vi "Main.vi"() -> ()   [LabVIEW 2018]
doc: "This Continuous Measurement sample project is based on the Queued Message Handler template.\n\nThe Event Handling Loop generates messages based on user interface actions.\n\nThe Message Handling Loop processes messages generated by the Event Handling Loop, or by other messages. There are also Acquisition and Logging message handling loop subVIs, and a chart updating loop."
uses:
  Settings/Settings.ctl
  Acquisition/Hardware Configuration.ctl
  Acquisition/Signal Type.ctl
  Logging/Logging Configuration.ctl
  controls/UI Data.ctl
  controls/UI State.ctl
  support/Message Queue/Enqueue Message (Single).vi
  controls/ExitGlobal.vi
  support/Message Queue/Enqueue Message (Array).vi
  <vilib>/Utility/error.llb/Error Cluster From Error Code.vi
  <vilib>/ErrorRing/Error Ring.xnode
  Acquisition/Acquisition.lvlib
  Logging/Logging.lvlib
  Settings/Settings.lvlib
  support/User Event - Stop/User Event - Stop.lvlib
  support/Message Queue/Message Queue.lvlib
  Settings/Settings Dialog.vi
panel:
  out "Data":waveform(dbl)[](graph)
  out "Zero run":bool
  in  "Zero run?":bool
  out "Max writing time to a file [min]":dbl
  out "Test time zero run [s]":dbl
  out "Test time [min]":dbl
  in  "Start":bool
  in  "Stop":bool
  in  "Settings":bool
  out "Status":string
  in  "Exit":bool
  out "Log File Offsite Path":path
  out "Project code":string
  out "Offsite storage?":bool
  out "Log File Path":path
  # "Continuous Measurement Data Logger"
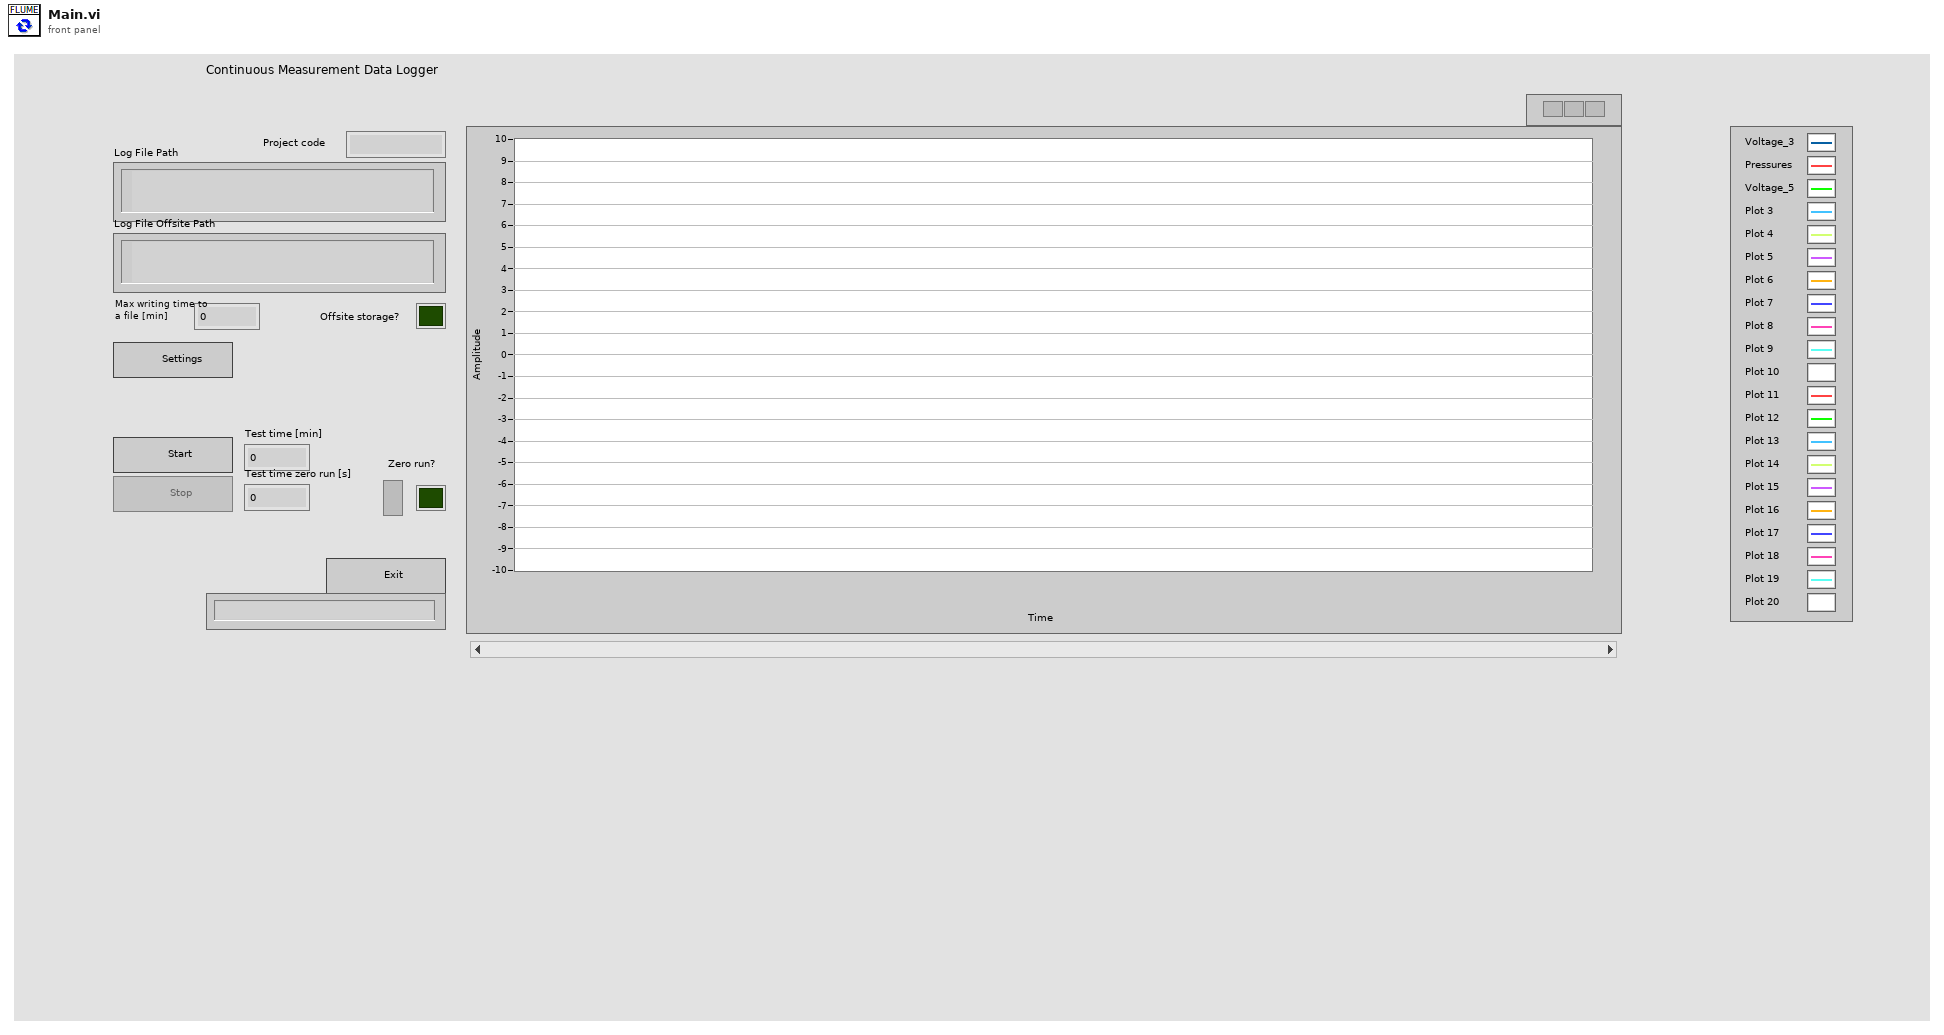
[diagram p1: front panel]
types:
  T1 = cluster{"Offsite storage?":bool, "Test time [s]":dbl, "Test time zero run [s] ":dbl, "Max writing time to a file [min]":dbl, "Zero run":bool}
  T2 = typedef "UI State.ctl" = enum16{"Idle", "Acquiring and Logging", "Waiting for Exit", "Waiting for Exit (Acq Stopped)", "Waiting for Exit (Log Stopped)", "Waiting for Stop", "Waiting for Stop (Acq Stopped)", "Waiting for Stop (Log Stopped)"}
  T3 = typedef "UI Data.ctl" = cluster{"Start Ref":refnum<vi>, "Stop Ref":refnum<vi>, "Settings Ref":refnum<vi>, "Exit Ref":refnum<vi>, "Status Ref":refnum<vi>, "Data Ref":refnum<vi>, "Zero run Ref":refnum<vi>}
  T4 = typedef "Settings.lvlib/Settings.ctl" = cluster{"Hardware Configuration":T5, "Logging Configuration":T7, "Timers":cluster{"Offsite storage?":bool, "Test time [s]":dbl, "Test time zero run [s] ":dbl, "Max writing time to a file [min]":dbl, "Zero run":bool}}
  T5 = typedef "Acquisition.lvlib/Hardware Configuration.ctl" = cluster{"DAQ1":string, "Signal Type 1":T6, "DAQ2":string, "Signal Type 2":T6, "DAQ3":string, "Signal Type 3":T6}
  T6 = typedef "Acquisition.lvlib/Signal Type.ctl" = enum16{"DAQ simulated", "Sine and square wave", "Sine wave"}
  T7 = typedef "Logging.lvlib/Logging Configuration.ctl" = cluster{"Log File Base Path":path, "TDMS File Reference":refnum<k34>, "Log File Offsite Path":path, "Project code":string, "Bin File Reference":refnum<k34>}
  T8 = typedef "Message Queue.lvlib/All Message Queues.ctl" = cluster{"UI":refnum<queue>, "Acquisition":refnum<queue>, "Logging":refnum<queue>, "Bin Logging":refnum<queue>, "Time":refnum<queue>}
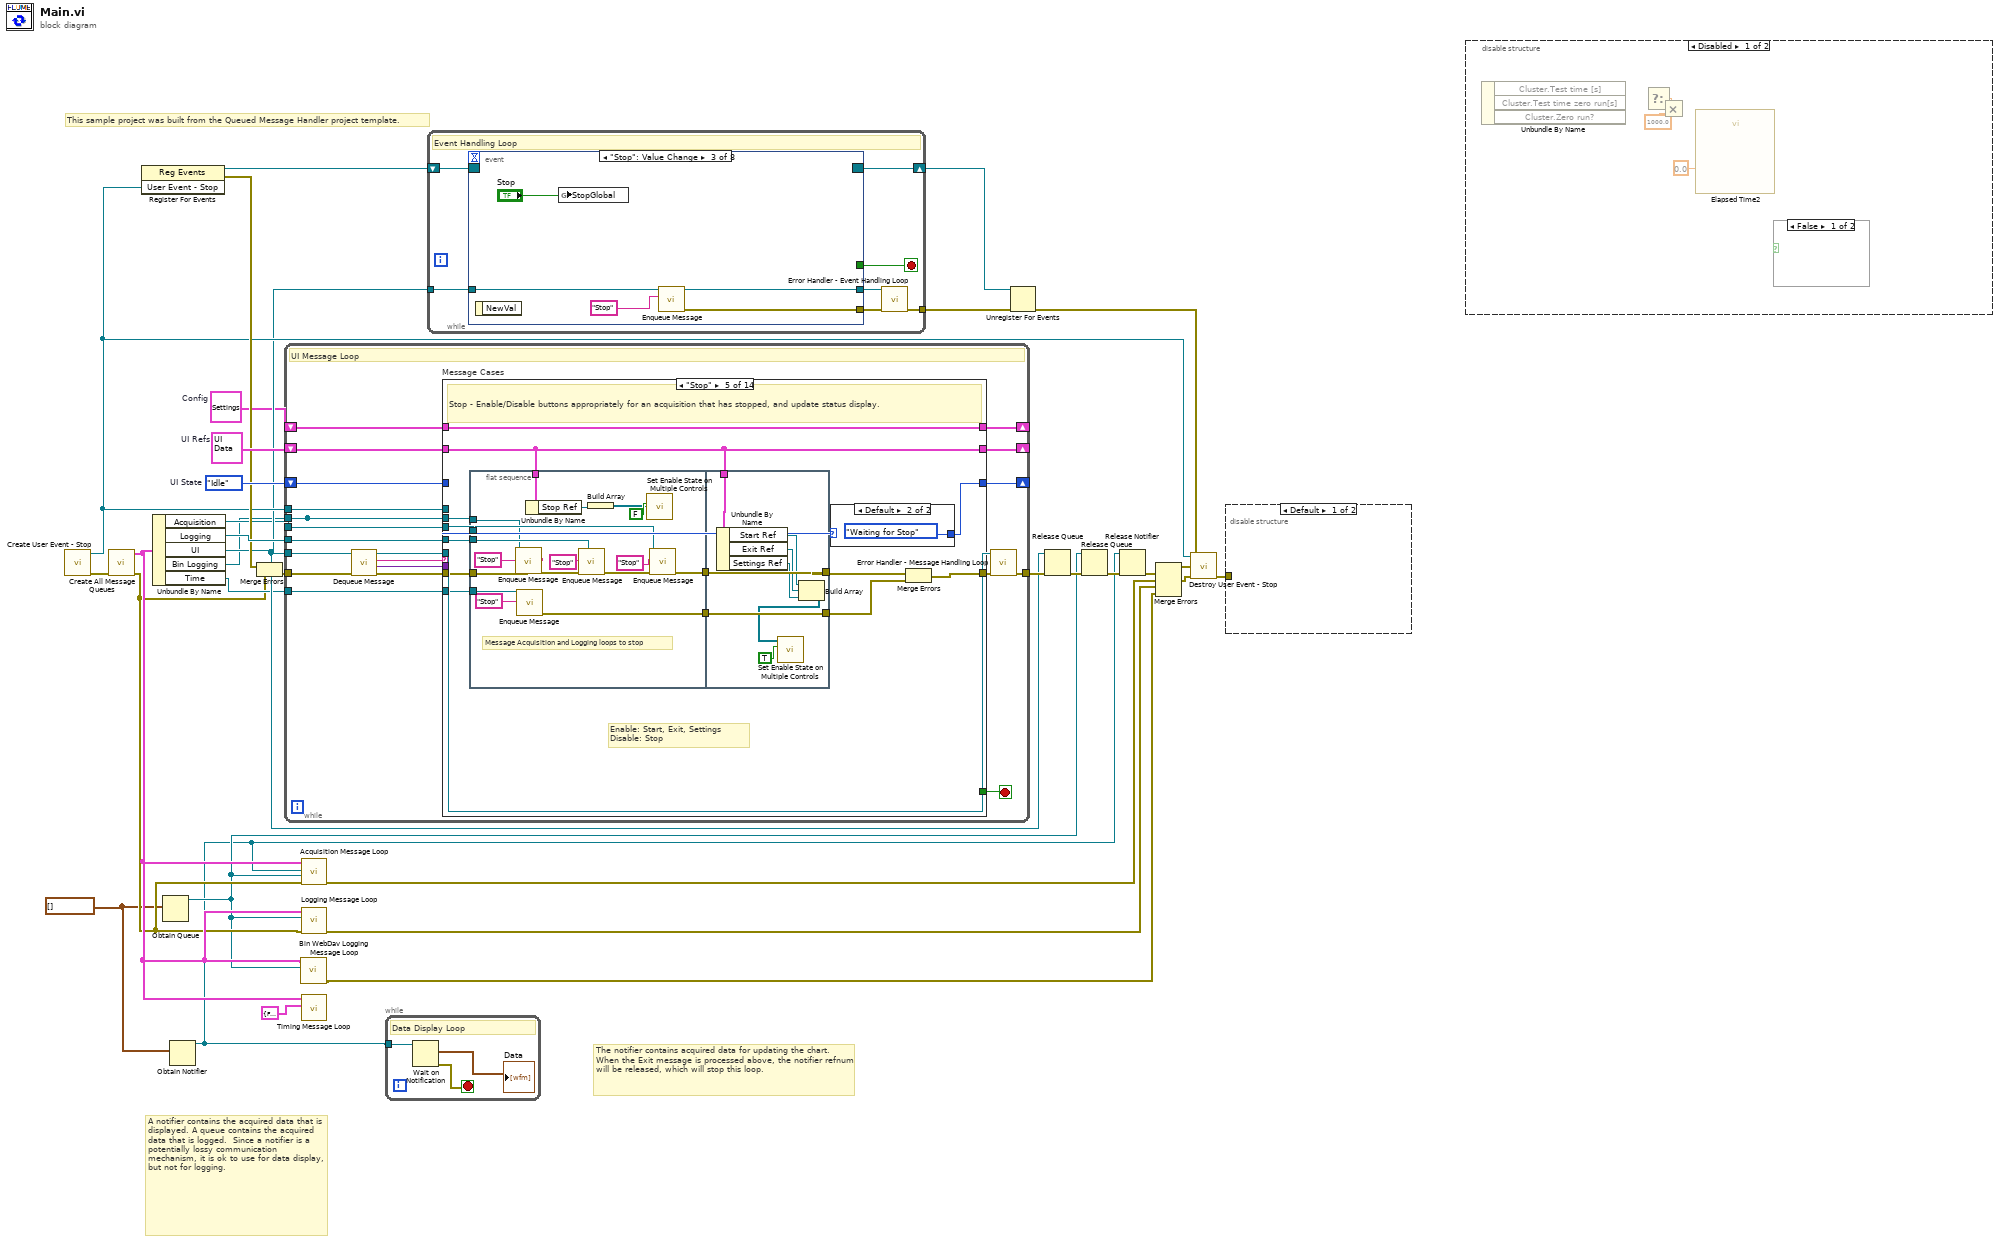
[diagram p0: block diagram]
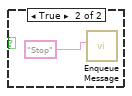
[diagram p2: hidden frame]
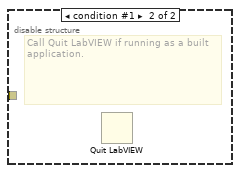
[diagram p4: hidden frame]
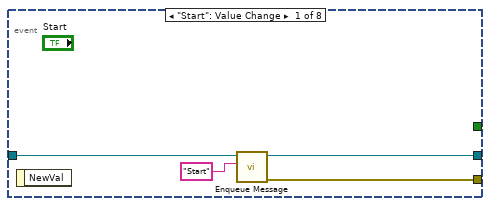
[diagram p5: hidden frame]
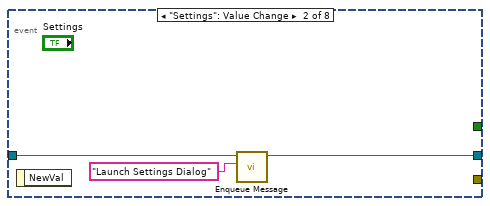
[diagram p6: hidden frame]
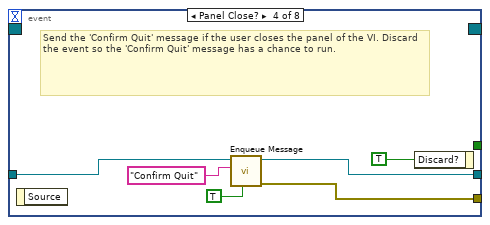
[diagram p7: hidden frame]
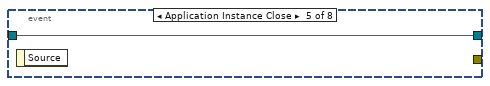
[diagram p8: hidden frame]
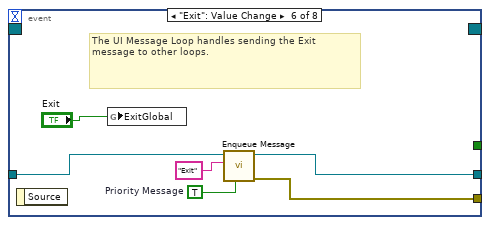
[diagram p9: hidden frame]
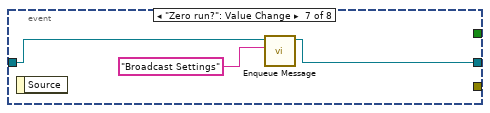
[diagram p10: hidden frame]
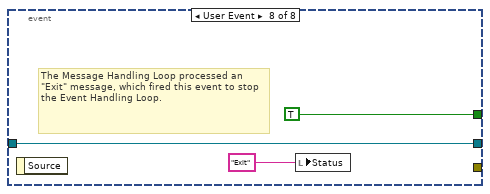
[diagram p11: hidden frame]
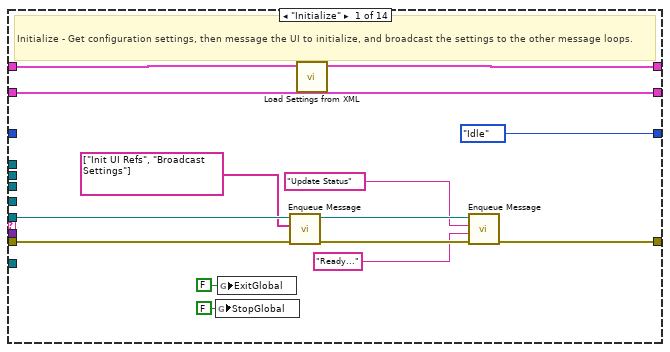
[diagram p12: hidden frame]
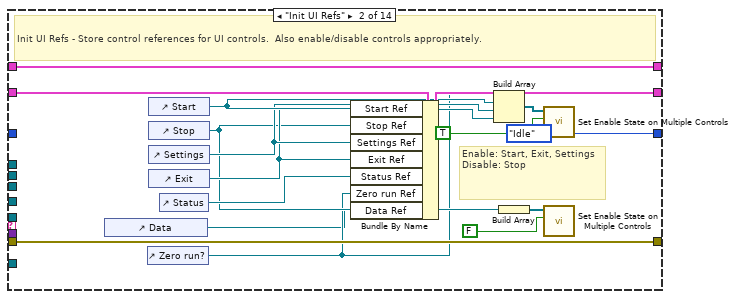
[diagram p13: hidden frame]
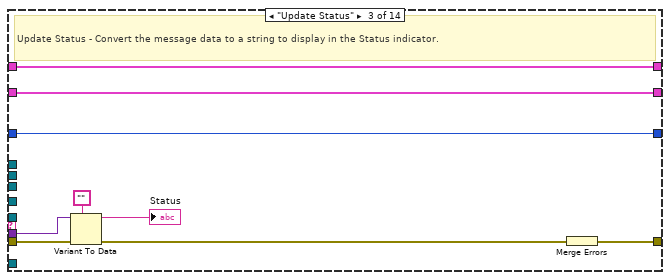
[diagram p14: hidden frame]
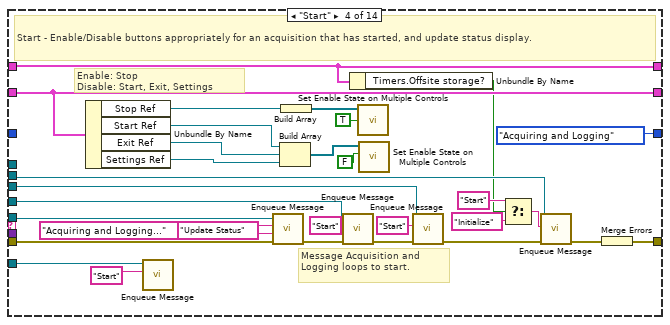
[diagram p15: hidden frame]
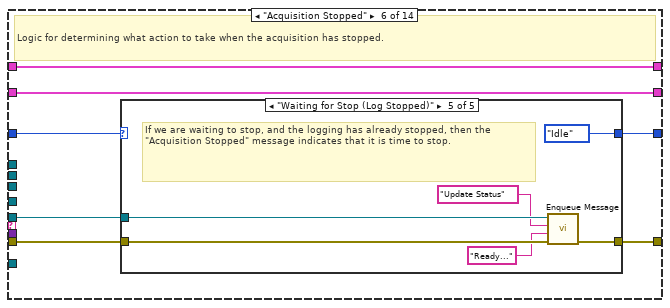
[diagram p17: hidden frame]
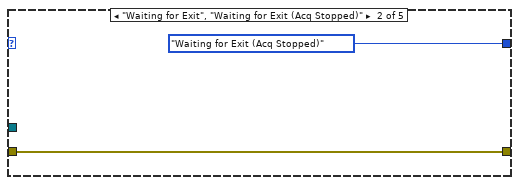
[diagram p19: hidden frame]
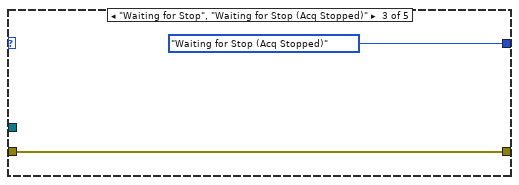
[diagram p20: hidden frame]
diagram:
  w2 = waveform(dbl)[] []
  w25 = UI_State."Idle"  # UI State
  w27 = T3 {"Start Ref"=refnum, "Stop Ref"=refnum, "Settings Ref"=refnum, "Exit Ref"=refnum, "Status Ref"=refnum, "Data Ref"=refnum, "Zero run Ref"=refnum}  # UI Refs
  w12 = T4 {"Hardware Configuration"={"DAQ1"="", "Signal Type 1"=enum."DAQ simulated", "DAQ2"="", "Signal Type 2"=enum."DAQ simulated", "DAQ3"="", "Signal Type 3"=enum."DAQ simulated"}, "Logging Configuration"={"Log File Base Path"=path "", "TDMS File Reference"=refnum, "Log File Offsite Path"=path "", "Project code"="", "Bin File Reference"=refnum}, "Timers"={"Offsite storage?"=FALSE, "Test time [s]"=10.0, "Test time zero run [s] "=180.0, "Max writing time to a file [min]"=30.0, "Zero run"=FALSE}}  # Config
  # "This sample project was built from the Queued Message Handler project template."
  # "A notifier contains the acquired data that is displayed. A queue contains the acquired data that is logged.  Since a notifier is a potentially lossy communication mechanism, it is ok to use for data display, but not for logging."
  # "The notifier contains acquired data for updating the chart. When the Exit message is processed above, the notifier refnum will be released, which will stop this loop."
  n1 = call "Create User Event - Stop.vi"() -> ("error out"=w29:errorcluster, "User Event - Stop"=w16:refnum<user-event>)  [unwired: 10 in]
  n2 = call "Create All Message Queues.vi"("error in (no error)"=w29) -> ("error out"=w4:errorcluster, "Message Queues out"=w5:T8)  [unwired: 9 in]
  n3 = register-events(w16) -> (reference out=w19:refnum<event-registration>, error out=w17:errorcluster)  [unwired: 2 in]
  n4 = Unbundle By Name(w5) -> ("Acquisition"=w14:refnum<queue>, "Logging"=w26:refnum<queue>, "UI"=w15:refnum<queue>, "Bin Logging"=w11:refnum<queue>, "Time"=w8:refnum<queue>)
  n5 = Obtain Queue(element data type=w2) -> (queue out=w3:refnum<queue>)  [unwired: 4 in, 2 out]
  n6 = Obtain Notifier(notification data type=w2) -> (notifier out=w1:refnum<notifier>)  [unwired: 3 in, 2 out]
  n7 = Merge Errors(w17, w4) -> (w18:errorcluster)
  n8 = while {
    tunnel: w15 -> [w38]
    tunnel: w16 -> [w50]
    shift-right: [w45] -> _
    shift-left: w12 -> [w34]
    shift-right: [w44] -> _
    shift-left: w27 -> [w32]
    tunnel: w14 -> [w43]
    tunnel: w26 -> [w37]
    shift-right: [w39] -> _
    shift-left: w25 -> [w40]
    tunnel: w18 -> [w49]
    tunnel: [w42] -> w31
    tunnel: w11 -> [w35]
    tunnel: [w35] -> _
    tunnel: w8 -> [w33]
    stop <- w51 stop-if-true
    # "UI Message Loop"
    n9 = call "Dequeue Message.vi"("error in (no error)"=w49, "Message Queue"=w38) -> ("error out"=w48:errorcluster, "Message Data"=w46:variant, "Message"=w47:string, "dup Message Queue"=w36:refnum<queue>)  [unwired: 6 in]
    n10 = case "Message Cases" shown="\"Stop\"" w47 {
      selector: w47 -> [_ _ _ _ _ _ _ _ _ _ _ _ _ w318]
      tunnel: w36 -> [w58 _ _ w102 _ w165 w190 _ w243 _ w265 _ _ _]
      tunnel: w48 -> [w57 w81 w89 w96 w134 w166 w191 w214 w245 w253 w264 w293 w316 _]
      tunnel: [w62 w81 w90 w104 w135 w163 w188 w212 w239 w256 w263 w309 w315 w317] -> w41
      tunnel: [_ _ _ _ _ _ _ _ _ _ _ TRUE _ _] -> w51
      tunnel: w46 -> [_ _ w88 _ _ _ _ _ _ w257 _ w302 _ _]
      tunnel: w50 -> [_ _ _ _ _ _ _ _ _ _ _ w310 _ _]
      tunnel: [w65 w69 w82 w95 w129 w162 w187 w216 w238 w252 w261 w300 w314 w321] -> w45
      tunnel: w34 -> [w54 w69 w82 w95 w129 w162 w187 w225 w246 w252 w261 w300 w314 w321]
      tunnel: w32 -> [w59 w80 w84 w119 w122 w168 w193 w235 w241 w260 w267 w308 w313 w320]
      tunnel: [w59 w78 w84 w119 w122 w168 w193 w235 w241 w260 w267 w308 w313 w320] -> w44
      tunnel: w43 -> [_ _ _ w103 w131 _ _ w234 _ _ _ w307 _ _]
      tunnel: w37 -> [_ _ _ w108 w133 _ _ w233 _ _ _ w306 _ _]
      tunnel: w40 -> [_ _ w83 _ w125 w167 w192 w232 w240 w255 w266 _ w312 w319]
      tunnel: [UI_State."Idle" ("UI State") UI_State."Idle" ("UI State") w83 UI_State."Acquiring and Logging" ("UI State") w130 w164 w189 w232 w240 w255 w262 UI_State."Idle" ("UI State") w312 w319] -> w39
      tunnel: w35 -> [_ _ _ w101 w128 _ _ w227 _ _ _ w299 _ _]
      tunnel: w33 -> [_ _ _ w99 w127 _ _ w224 _ _ _ w298 _ _]
      frame "Initialize" {
        # "Initialize - Get configuration settings, then message the UI to initialize, and broadcast the settings to the other message loops."
        n11 = global write "ExitGlobal.vi" "StopGlobal"(FALSE ("ExitGlobal")) -> ()
        n12 = global write "ExitGlobal.vi" "ExitGlobal"(FALSE ("ExitGlobal")) -> ()
        n13 = call-poly "Enqueue Message.vi"("error in (no error)"=w57, "Message Array"=string[] ["Init UI Refs", "Broadcast Settings"], "Message Queue"=w58) -> ("error out"=w64:errorcluster, "dup Message Queue"=w63:refnum<queue>)  [unwired: 7 in]
        n14 = call "Load Settings from XML.vi"("Settings in"=w54) -> ("Settings out"=w65:T4)  [unwired: 9 in, 1 out]
        n15 = call-poly "Enqueue Message.vi"("error in (no error)"=w64, "Message Data"="Ready..." ("Ready..."), "Message"="Update Status", "Message Queue"=w63) -> ("error out"=w62:errorcluster)  [unwired: 6 in, 1 out]
      }
      frame "Init UI Refs" {
        # "Enable: Start, Exit, Settings\nDisable: Stop"
        # "Init UI Refs - Store control references for UI controls.  Also enable/disable controls appropriately."
        n16 = control-ref of="Data"() -> (w66:refnum<vi>)
        n17 = control-ref of="Zero run?"() -> (w67:refnum<vi>)
        n18 = control-ref of="Start"() -> (w73:refnum<vi>)
        n19 = control-ref of="Stop"() -> (w68:refnum<vi>)
        n20 = control-ref of="Settings"() -> (w72:refnum<vi>)
        n21 = control-ref of="Exit"() -> (w71:refnum<vi>)
        n22 = control-ref of="Status"() -> (w79:refnum<vi>)
        n23 = Bundle By Name(cluster=w80, "Start Ref"=w73, "Stop Ref"=w68, "Settings Ref"=w72, "Exit Ref"=w71, "Status Ref"=w79, "Zero run Ref"=w67, "Data Ref"=w66) -> (w78:T3)
        n24 = Build Array(w67, w73, w72, w71) -> (w76:refnum<vi>[])
        n25 = Build Array(w68) -> (w75:refnum<vi>[])
        n26 = call "Set Enable State on Multiple Controls.vi"("Enable?"=TRUE, "Controls"=w76) -> ()  [unwired: 10 in]
        n27 = call "Set Enable State on Multiple Controls.vi"("Enable?"=FALSE, "Controls"=w75) -> ()  [unwired: 10 in]
      }
      frame "Update Status" {
        # "Update Status - Convert the message data to a string to display in the Status indicator."
        n28 = Variant To Data(error in=w89, type="", Variant=w88) -> (data=→"Status":string, error out=w86:errorcluster)
        n29 = Merge Errors(w86) -> (w90:errorcluster)
      }
      frame "Start" {
        # "Message Acquisition and Logging loops to start."
        # "Enable: Stop\nDisable: Start, Exit, Settings"
        # "Start - Enable/Disable buttons appropriately for an acquisition that has started, and update status display."
        n30 = Unbundle By Name(w119) -> ("Stop Ref"=w114:refnum<vi>, "Start Ref"=w113:refnum<vi>, "Exit Ref"=w112:refnum<vi>, "Settings Ref"=w111:refnum<vi>)
        n31 = call-poly "Enqueue Message.vi"("Message"="Start", "Message Queue"=w99) -> ()  [unwired: 8 in, 2 out]
        n32 = call-poly "Enqueue Message.vi"("error in (no error)"=w96, "Message Data"="Acquiring and Logging..." ("Acquiring and Logging..."), "Message"="Update Status", "Message Queue"=w102) -> ("error out"=w110:errorcluster)  [unwired: 6 in, 1 out]
        n33 = Build Array(w113, w112, w111) -> (w117:refnum<vi>[])
        n34 = Build Array(w114) -> (w116:refnum<vi>[])
        n35 = call-poly "Enqueue Message.vi"("error in (no error)"=w110, "Message"="Start", "Message Queue"=w108) -> ("error out"=w105:errorcluster)  [unwired: 7 in, 1 out]
        n36 = Unbundle By Name(w95) -> ("Timers.Offsite storage?"=w92:bool)
        n37 = call "Set Enable State on Multiple Controls.vi"("Enable?"=TRUE, "Controls"=w116) -> ()  [unwired: 10 in]
        n38 = call "Set Enable State on Multiple Controls.vi"("Enable?"=FALSE, "Controls"=w117) -> ()  [unwired: 10 in]
        n39 = call-poly "Enqueue Message.vi"("error in (no error)"=w105, "Message"="Start", "Message Queue"=w103) -> ("error out"=w98:errorcluster)  [unwired: 7 in, 1 out]
        n40 = Select(t="Start" ("Message"), s=w92, f="Initialize") -> (s? t:f=w91:string)
        n41 = call-poly "Enqueue Message.vi"("error in (no error)"=w98, "Message"=w91, "Message Queue"=w101) -> ("error out"=w97:errorcluster)  [unwired: 7 in, 1 out]
        n42 = Merge Errors(w97) -> (w104:errorcluster)
      }
      frame "Stop" {
        # "Enable: Start, Exit, Settings\nDisable: Stop"
        # "Stop - Enable/Disable buttons appropriately for an acquisition that has stopped, and update status display."
        n43 = flat-sequence {
          tunnel: w134 -> [w151]
          tunnel: w133 -> [w149]
          tunnel: w131 -> [w146]
          tunnel: w128 -> [w143]
          tunnel: w127 -> [w142]
          tunnel: [w147] -> w124
          tunnel: [w140] -> w123
          tunnel: w122 -> [w138]
          tunnel: [w158] -> w126
          tunnel: [w159] -> w132
          tunnel: w124 -> [w159]
          tunnel: w123 -> [w158]
          tunnel: w122 -> [w155]
          frame #0 {
            # "Message Acquisition and Logging loops to stop"
            n44 = call-poly "Enqueue Message.vi"("Message"="Stop", "Message Queue"=w143) -> ()  [unwired: 8 in, 2 out]
            n45 = call-poly "Enqueue Message.vi"("Message"="Stop", "Message Queue"=w142) -> ("error out"=w140:errorcluster)  [unwired: 8 in, 1 out]
            n46 = Unbundle By Name(w138) -> ("Stop Ref"=w137:refnum<vi>)
            n47 = call-poly "Enqueue Message.vi"("error in (no error)"=w151, "Message"="Stop", "Message Queue"=w149) -> ("error out"=w148:errorcluster)  [unwired: 7 in, 1 out]
            n48 = Build Array(w137) -> (w136:refnum<vi>[])
            n49 = call "Set Enable State on Multiple Controls.vi"("Enable?"=FALSE, "Controls"=w136) -> ()  [unwired: 10 in]
            n50 = call-poly "Enqueue Message.vi"("error in (no error)"=w148, "Message"="Stop", "Message Queue"=w146) -> ("error out"=w147:errorcluster)  [unwired: 7 in, 1 out]
          }
          frame #1 {
            n51 = Unbundle By Name(w155) -> ("Start Ref"=w154:refnum<vi>, "Exit Ref"=w153:refnum<vi>, "Settings Ref"=w152:refnum<vi>)
            n52 = Build Array(w154, w153, w152) -> (w157:refnum<vi>[])
            n53 = call "Set Enable State on Multiple Controls.vi"("Enable?"=TRUE, "Controls"=w157) -> ()  [unwired: 10 in]
          }
        }
        n54 = case shown="Default" w125 {
          selector: w125 -> [w160 _]
          tunnel: [w160 UI_State."Waiting for Stop" ("UI State")] -> w130
          frame "Waiting for Exit" {
          }
          frame Default {
          }
        }
        n55 = Merge Errors(w132, w126) -> (w135:errorcluster)
      }
      frame "Acquisition Stopped" {
        # "Logic for determining what action to take when the acquisition has stopped."
        n56 = case shown="\"Waiting for Stop (Log Stopped)\"" w167 {
          selector: w167 -> [w170 _ _ _ _]
          tunnel: w166 -> [w169 w172 w174 w180 w186]
          tunnel: w165 -> [_ _ _ w178 w183]
          tunnel: [w170 UI_State."Waiting for Exit (Acq Stopped)" ("UI State") UI_State."Waiting for Stop (Acq Stopped)" ("UI State") UI_State."Idle" ("UI State") UI_State."Idle" ("UI State")] -> w164
          tunnel: [w169 w172 w174 w179 w184] -> w163
          frame Default {
          }
          frame "Waiting for Exit", "Waiting for Exit (Acq Stopped)" {
          }
          frame "Waiting for Stop", "Waiting for Stop (Acq Stopped)" {
          }
          frame "Waiting for Exit (Log Stopped)" {
            # "If we are waiting to exit, and the logging has already stopped, then the \"Acquisition Stopped\" message indicates that it is time to exit."
            n57 = call-poly "Enqueue Message.vi"("Priority Message? (F)"=TRUE, "error in (no error)"=w180, "Message"="Exit", "Message Queue"=w178) -> ("error out"=w179:errorcluster)  [unwired: 6 in, 1 out]
          }
          frame "Waiting for Stop (Log Stopped)" {
            # "If we are waiting to stop, and the logging has already stopped, then the \"Acquisition Stopped\" message indicates that it is time to stop."
            n58 = call-poly "Enqueue Message.vi"("error in (no error)"=w186, "Message Data"="Ready..." ("Ready..."), "Message"="Update Status", "Message Queue"=w183) -> ("error out"=w184:errorcluster)  [unwired: 6 in, 1 out]
          }
        }
      }
      frame "Logging Stopped" {
        # "Logic for determining what action to take when the logging has stopped."
        n59 = case shown="Default" w192 {
          selector: w192 -> [w195 _ _ _ _]
          tunnel: w191 -> [w194 w197 w199 w205 w208]
          tunnel: w190 -> [_ _ _ w203 w207]
          tunnel: [w195 UI_State."Waiting for Exit (Log Stopped)" ("UI State") UI_State."Waiting for Stop (Log Stopped)" ("UI State") UI_State."Idle" ("UI State") UI_State."Idle" ("UI State")] -> w189
          tunnel: [w194 w197 w199 w204 w206] -> w188
          frame Default {
          }
          frame "Waiting for Exit", "Waiting for Exit (Log Stopped)" {
          }
          frame "Waiting for Stop", "Waiting for Stop (Log Stopped)" {
          }
          frame "Waiting for Exit (Acq Stopped)" {
            # "If we are waiting to exit, and the acquisition has already stopped, then the \"Logging Stopped\" message indicates that it is time to exit."
            n60 = call-poly "Enqueue Message.vi"("Priority Message? (F)"=TRUE, "error in (no error)"=w205, "Message"="Exit", "Message Queue"=w203) -> ("error out"=w204:errorcluster)  [unwired: 6 in, 1 out]
          }
          frame "Waiting for Stop (Acq Stopped)" {
            # "If we are waiting to stop, and the acquisition has already stopped, then the \"Logging Stopped\" message indicates that it is time to stop."
            n61 = call-poly "Enqueue Message.vi"("error in (no error)"=w208, "Message Data"="Ready..." ("Ready..."), "Message"="Update Status", "Message Queue"=w207) -> ("error out"=w206:errorcluster)  [unwired: 6 in, 1 out]
          }
        }
      }
      frame "Broadcast settings" {
        w223 = "Update Settings" ("Message")
        # "Broadcast settings - Send the 'Update Settings' message to the Logging and Acquisition message loops."
        n62 = Bundle By Name(cluster=w225, "Timers.Zero run"="Zero run?") -> (w216:T4)
        n63 = Unbundle By Name(w216) -> ("Hardware Configuration"=w236:T5, "Logging Configuration"=w217:T7, "Timers"=w222:T1)
        n64 = Unbundle By Name(w222) -> ("Max writing time to a file [min]"=→"Max writing time to a file [min]":dbl, "Offsite storage?"=→"Offsite storage?":bool, "Test time [s]"=→"Test time [min]":dbl, "Test time zero run [s]"=→"Test time zero run [s]":dbl)
        n65 = Unbundle By Name(w217) -> ("Log File Base Path"=→"Log File Path":path, "Log File Offsite Path"=→"Log File Offsite Path":path, "Project code"=→"Project code":string)
        n66 = call-poly "Enqueue Message.vi"("error in (no error)"=w214, "Message Data"=w217, "Message"=w223, "Message Queue"=w227) -> ("error out"=w215:errorcluster)  [unwired: 6 in, 1 out]
        n67 = Unbundle By Name(w216) -> ("Timers"=w220:T1)
        n68 = call-poly "Enqueue Message.vi"("error in (no error)"=w215, "Message Data"=w236, "Message"=w223, "Message Queue"=w234) -> ("error out"=w237:errorcluster)  [unwired: 6 in, 1 out]
        n69 = call-poly "Enqueue Message.vi"("error in (no error)"=w237, "Message Data"=w217, "Message"=w223, "Message Queue"=w233) -> ("error out"=w213:errorcluster)  [unwired: 6 in, 1 out]
        n70 = call-poly "Enqueue Message.vi"("error in (no error)"=w213, "Message Data"=w220, "Message"=w223, "Message Queue"=w224) -> ("error out"=w212:errorcluster)  [unwired: 6 in, 1 out]
        "Zero run" <- "Zero run?"
      }
      frame "Launch Settings Dialog" {
        # "Launch Settings Dialog - Launch the Settings Dialog when the user clicks the 'Settings' button."
        n71 = call-by-ref "?"("error in (no error)"=w245, "Settings in"=w246) -> ("error out"=w242:errorcluster, "Cancelled?"=w244:bool, "Settings out"=w238:T4)  [unwired: 8 in, 3 out]
        n72 = case shown="False" w244 {
          tunnel: w243 -> [w250 _]
          tunnel: w242 -> [w249 w251]
          tunnel: [w248 w251] -> w239
          frame False {
            n73 = call-poly "Enqueue Message.vi"("error in (no error)"=w249, "Message"="Broadcast Settings", "Message Queue"=w250) -> ("error out"=w248:errorcluster)  [unwired: 7 in, 1 out]
          }
          frame True {
          }
        }
      }
      frame "Error" {
        # "Error - Display an error dialog. This message is sent by the \"Error Handler\" VIs at the end of other loops in this application."
        n74 = Variant To Data(error in=w253, type=errorcluster {"status"=FALSE, "code"=0, "source"=""} ("error constant"), Variant=w257) -> (data=w254:errorcluster, error out=w258:errorcluster)
        n75 = call <vilib>:"Simple Error Handler.vi"("error in (no error)"=w254) -> ()  [unwired: 4 in, 5 out]
        n76 = Merge Errors(w258) -> (w256:errorcluster)
      }
      frame "Confirm Quit" {
        # "Confirm Quit - Message that can confirm whether or not the user wants to exit the application."
        n77 = case shown="\"Acquiring and Logging\"" w266 {
          tunnel: w265 -> [w273 w277]
          tunnel: w264 -> [w272 w276]
          tunnel: [w271 w275] -> w263
          tunnel: [UI_State."Idle" ("UI State") w274] -> w262
          frame Default {
            # "If 'Confirm Quit' comes in while the system is idle, there is no need for a confirmation message."
            n78 = call-poly "Enqueue Message.vi"("Priority Message? (F)"=TRUE, "error in (no error)"=w272, "Message"="Exit", "Message Queue"=w273) -> ("error out"=w271:errorcluster)  [unwired: 6 in, 1 out]
          }
          frame "Acquiring and Logging" {
            n79 = Two Button Dialog(message="Are you sure you want to quit while the acquisition is running?" ("Confirm Quit Message"), 1:"No" ("No"), 2:"Yes" ("Yes")) -> (T button?=w278:bool)
            n80 = case shown="True" w278 {
              tunnel: w277 -> [_ w287]
              tunnel: w276 -> [w283 w288]
              tunnel: [w283 w286] -> w275
              tunnel: [UI_State."Acquiring and Logging" ("UI State") UI_State."Waiting for Exit" ("UI State")] -> w274
              frame False {
                # "User did not want to quit."
              }
              frame True {
                n81 = call-poly "Enqueue Message.vi"("error in (no error)"=w288, "Message"="Stop", "Message Queue"=w287) -> ("error out"=w286:errorcluster)  [unwired: 7 in, 1 out]
              }
            }
          }
        }
      }
      frame "Exit" {
        w295 = "Exit" ("Message")
        # "Popup an error dialog if 'Exit' was called as a result of an error."
        # "Stop the VI"
        # "Exit - Send Exit messages to the Acquisition and Logging loops, and fire the user event to stop the Event Handling Loop."
        n82 = Variant To Data(type=errorcluster {"status"=FALSE, "code"=0, "source"=""} ("error constant"), Variant=w302) -> (data=w301:errorcluster)  [unwired: 1 in, 1 out]
        n83 = call-poly "Enqueue Message.vi"("Priority Message? (F)"=TRUE, "error in (no error)"=w293, "Message"=w295, "Message Queue"=w307) -> ("error out"=w292:errorcluster)  [unwired: 6 in, 1 out]
        n84 = call <vilib>:"Simple Error Handler.vi"("error in (no error)"=w301) -> ()  [unwired: 4 in, 5 out]
        n85 = call-poly "Enqueue Message.vi"("Priority Message? (F)"=TRUE, "error in (no error)"=w292, "Message"=w295, "Message Queue"=w306) -> ("error out"=w291:errorcluster)  [unwired: 6 in, 1 out]
        n86 = call-poly "Enqueue Message.vi"("Priority Message? (F)"=TRUE, "error in (no error)"=w291, "Message"=w295, "Message Queue"=w299) -> ("error out"=w290:errorcluster)  [unwired: 6 in, 1 out]
        n87 = call-poly "Enqueue Message.vi"("Priority Message? (F)"=TRUE, "error in (no error)"=w290, "Message"=w295, "Message Queue"=w298) -> ("error out"=w289:errorcluster)  [unwired: 6 in, 1 out]
        n88 = call "Fire User Event - Stop.vi"("error in (no error)"=w289, "User Event - Stop"=w310) -> ("error out"=w309:errorcluster)  [unwired: 9 in]
      }
      frame "---Copy This Frame---" {
        # "Duplicate this frame when creating new messages.  Change this comment in the duplicated frame to describe this message."
        n89 = Merge Errors(w316) -> (w315:errorcluster)
      }
      frame Default {
        # "'Default' case only runs if there is a message that isn't defined in any of the other cases.  Output a programming error."
        n90 = xnode "Error Ring"("parameter 0"=w318) -> ("error out"=w317:errorcluster)
      }
    }
    n91 = call "Error Handler - Message Handling Loop.vi"("error in (no error)"=w41, "Message Queue"=w36) -> ("dup error in"=w42:errorcluster)  [unwired: 8 in, 1 out]
  }
  n92 = call "Bin WebDav Logging Message Loop.vi"("Data Queue"=w3, "Message Queues"=w5) -> ("error out"=w6:errorcluster)  [unwired: 9 in]
  n93 = call "Acquisition Message Loop.vi"("error in (no error)"=w4, "Data Queue"=w3, "Data Notifier"=w1, "Message Queues"=w5) -> ("error out"=w7:errorcluster)  [unwired: 7 in]
  n94 = call "Logging Message Loop.vi"("error in (no error)"=w4, "Data Queue"=w3, "Message Queues"=w5) -> ("error out"=w10:errorcluster)  [unwired: 8 in]
  n95 = call "Timing Message Loop.vi"("Timers"=T1 {"Offsite storage?"=FALSE, "Test time [s]"=0.0, "Test time zero run [s] "=0.0, "Max writing time to a file [min]"=0.0, "Zero run"=FALSE}, "Message Queues"=w5) -> ()  [unwired: 9 in, 1 out]
  n96 = while "Data Display Loop" {
    tunnel: w1 -> [w331]
    stop <- w330 stop-if-true
    # "Data Display Loop"
    n97 = Wait on Notification(notifier=w331) -> (notification=→"Data":waveform(dbl)[], error out=w330:errorcluster)  [unwired: 3 in, 2 out]
  }
  n98 = while {
    tunnel: w15 -> [w337]
    tunnel: [w334] -> w30
    shift-right: [w336] -> w28
    shift-left: w19 -> [w338]
    stop <- w335 stop-if-true
    # "Event Handling Loop"
    n99 = event shown="[2] \"Stop\": Value Change" {
      selector: w338 -> [_ _ _ _ _ _ _ _]
      dyn-events: [_ _ _ _ _ _ _ _] -> w336
      timeout: _ -> [_ _ _ _ _ _ _ _]
      tunnel: [_ _ _ _ _ _ _ TRUE ("Discard?")] -> w335
      tunnel: w337 -> [w342 w344 w349 w354 w357 w360 w365 w367]
      tunnel: [w340 _ w348 w352 _ w363 _ _] -> w333
      tunnel: [w339 w343 w347 w353 w357 w359 w364 w367] -> w332
      event "Start": Value Change {
        n100 = event-data() -> ()  [unwired: 1 in, 1 out]
        n101 = call-poly "Enqueue Message.vi"("Message"="Start", "Message Queue"=w342) -> ("error out"=w340:errorcluster, "dup Message Queue"=w339:refnum<queue>)  [unwired: 8 in]
      }
      event "Settings": Value Change {
        n102 = event-data() -> ()  [unwired: 1 in, 1 out]
        n103 = call-poly "Enqueue Message.vi"("Message"="Launch Settings Dialog", "Message Queue"=w344) -> ("dup Message Queue"=w343:refnum<queue>)  [unwired: 8 in, 1 out]
      }
      event "Stop": Value Change {
        n104 = event-data() -> ()  [unwired: 1 in, 1 out]
        n105 = global write "ExitGlobal.vi" "StopGlobal"("Stop") -> ()
        n106 = call-poly "Enqueue Message.vi"("Message"="Stop", "Message Queue"=w349) -> ("error out"=w348:errorcluster, "dup Message Queue"=w347:refnum<queue>)  [unwired: 8 in]
      }
      event Panel Close? {
        # "Send the 'Confirm Quit' message if the user closes the panel of the VI. Discard the event so the 'Confirm Quit' message has a chance to run."
        n107 = event-data() -> ()  [unwired: 1 in, 1 out]
        n108 = call-poly "Enqueue Message.vi"("Priority Message? (F)"=TRUE, "Message"="Confirm Quit", "Message Queue"=w354) -> ("error out"=w352:errorcluster, "dup Message Queue"=w353:refnum<queue>)  [unwired: 7 in]
        n109 = event-data("Discard?"=TRUE) -> ()  [unwired: 1 in, 1 out]
      }
      event Application Instance Close {
        n110 = event-data() -> ()  [unwired: 1 in, 1 out]
      }
      event "Exit": Value Change {
        w361 = TRUE  # Priority Message
        # "The UI Message Loop handles sending the Exit message to other loops."
        n111 = event-data() -> ()  [unwired: 1 in, 1 out]
        n112 = global write "ExitGlobal.vi" "ExitGlobal"("Exit") -> ()
        n113 = call-poly "Enqueue Message.vi"("Priority Message? (F)"=w361, "Message"="Exit", "Message Queue"=w360) -> ("error out"=w363:errorcluster, "dup Message Queue"=w359:refnum<queue>)  [unwired: 7 in]
      }
      event "Zero run?": Value Change {
        n114 = event-data() -> ()  [unwired: 1 in, 1 out]
        n115 = call-poly "Enqueue Message.vi"("Message"="Broadcast Settings", "Message Queue"=w365) -> ("dup Message Queue"=w364:refnum<queue>)  [unwired: 8 in, 1 out]
      }
      event User Event {
        # "The Message Handling Loop processed an \"Exit\" message, which fired this event to stop the Event Handling Loop."
        n116 = event-data() -> ()  [unwired: 1 in, 1 out]
        n117 = local write "Status"("Exit" ("Exit String")) -> ()
      }
    }
    n118 = call "Error Handler - Event Handling Loop.vi"("error in (no error)"=w333, "Message Queue"=w332) -> ("dup error in"=w334:errorcluster)  [unwired: 8 in, 1 out]
  }
  n119 = Unregister For Events(event registration refnum=w28, error in=w30) -> (error out=w13:errorcluster)
  n120 = Release Queue(queue=w15, error in (no error)=w31) -> (error out=w22:errorcluster)  [unwired: 1 in, 2 out]
  n121 = Release Queue(queue=w3, error in (no error)=w22) -> (error out=w21:errorcluster)  [unwired: 1 in, 2 out]
  n122 = Release Notifier(notifier=w1, error in (no error)=w21) -> (error out=w20:errorcluster)  [unwired: 1 in, 2 out]
  n123 = Merge Errors(w13, w20, w7, w10, w6) -> (w24:errorcluster)
  n124 = call "Destroy User Event - Stop.vi"("error in (no error)"=w24, "User Event - Stop"=w16) -> ("error out"=w23:errorcluster)  [unwired: 9 in]
  n125 = disable-structure shown="Default" {
    disable-tunnel: w23 -> [_ _]
    frame condition #0 (active) {
    }
    frame condition #1 {
      # "Call Quit LabVIEW if running as a built application."
      n126 = Quit LabVIEW() -> ()  [unwired: 1 in]
    }
  }
  n127 = disable-structure shown="Disabled" {
    frame Disabled {
      n128 = Unbundle By Name() -> ()  [unwired: 1 in, 3 out]
      n129 = Select() -> (s? t:f=w372:dbl)  [unwired: 3 in]
      n130 = Multiply(x=w372, y=1000.0) -> ()  [unwired: 1 out]
      n131 = call "Elapsed Time2"("Set Start Time (s)"=0.0) -> ()  [unwired: 11 in, 8 out]
      n132 = case shown="False" {
        selector: _ -> [_ _]
        frame False {
        }
        frame True {
          n133 = call-poly "Enqueue Message.vi"("Message"="Stop") -> ()  [unwired: 9 in, 2 out]
        }
      }
    }
    frame Enabled {
    }
  }
